vi "CSMStandApp.vi"() -> ()   [LabVIEW 2020, in "CSMStand-Engine(Lite).lvlib"]
doc: "------------- lvcsm -------------\n[CSMStates]\nItem 0 = \"Event Structure\"\nItem 1 = \"Idle\"\nItem 2 = \"CSM Documentation\"\nItem 3 = \"Error Handler\"\nItem 4 = \"VI Reference\"\nItem 5 = \"Critical Error\"\nItem 6 = \"Target Timeout Error\"\nItem 7 = \"Target Error\"\nItem 8 = \"Async Response\"\nItem 9 = \"Response\"\nItem 10 = \"Async Message Posted\"\nItem 11 = \"Initialize Core Data\"\nItem 12 = \"Exit\"\nItem 13 = \"Data: Initialize\"\nItem 14 = \"Data: Get Configuration\"\nItem 15 = \"Data: Get Internal Data\"\nItem 16 = \"Data: Set Configuration\"\nItem 17 = \"Data: Cleanup\"\nItem 18 = \"Events: Register\"\nItem 19 = \"Events: Unregister\"\nItem 20 = \"UI: Initialize\"\nItem 21 = \"UI: Cursor Set\"\nItem 22 = \"UI: Front Panel State\"\nItem 23 = \"UI: Insert CSMStand OI\"\nItem 24 = \"UI: Start CSMStand Engine Behind\"\nItem 25 = \"UI: Show Version Dialog\"\nItem 26 = \"UI: Update Title\"\nItem 27 = \"Macro: Initialize\"\nItem 28 = \"Macro: Exit\"\nItem 29 = \"API: Load Script File\"\nItem 30 = \"API: Unload Sequence File\"\nItem 31 = \"API: Information\"\nItem 32 = \"API: Settings\"\n\n[CSMStatus]\nItem 0 = \"Error Occurred@Error Handler\""
uses:
  f71e1bc3-10f1-4d1d-8987-c57c60744672.vi
  5479b9e0-3b99-47d2-9fb2-6b1a6c6fc50e.vi
  48aabd89-37f9-4145-9c04-d0fd28b441f4.vi
  35608a63-0d23-4e3c-87b1-9318b6aa47ba.vi
  1ae25337-ae93-478f-b23d-9afa4476f43f.vi
  <userlib>/_NEVSTOP/Communicable State Machine(CSM)/AdvanceAPI/CSM - Revert Arguments-Safe String.vi
  <userlib>/_NEVSTOP/Communicable State Machine(CSM)/AdvanceAPI/CSM - Break Down Multiple States String.vi
  <userlib>/_NEVSTOP/Communicable State Machine(CSM)/AdvanceAPI/CSM - Compact Multiple States.vi
  <userlib>/_NEVSTOP/Communicable State Machine(CSM)/AdvanceAPI/CSM - Keywords.vi
  <userlib>/_NEVSTOP/Communicable State Machine(CSM)/_Shared/Trim Single-line Text.vi
  <userlib>/_NEVSTOP/Communicable State Machine(CSM)/addons/API-String-Arugments-Support/_Support/Query Data as API String Arguments(variant).vi
  <userlib>/_NEVSTOP/Communicable State Machine(CSM)/addons/API-String-Arugments-Support/_Support/Convert API String Arguments to Data(variant).vi
  UI/ExecutionView(CSM).vi
  Engine/Engine(CSM).vi
  UI/VersionDialog(CSM).vi
  <userlib>/NEVSTOP-Programming-Palette/Dialog & Interface/Fit VI window to Caller Center_nevstop.vi
  <userlib>/_NEVSTOP/Communicable State Machine(CSM)/addons/API-String-Arugments-Support/_Support/Data To API String Arguments.vi
  <userlib>/_NEVSTOP/Communicable State Machine(CSM)/addons/MassData-Parameter/_support/FGV-MassData(lvlibp).vi
  CSMStand-Engine(Lite).lvlib
  <userlib>/_NEVSTOP/Communicable State Machine(CSM)/Communicable State Machine.lvlib
  <userlib>/_NEVSTOP/Communicable State Machine(CSM)/_tool/_ui/csm-ui-support.lvlib
  <userlib>/_NEVSTOP/Communicable State Machine(CSM)/addons/API-String-Arugments-Support/API String Arguments Support.lvlib
  <userlib>/_NEVSTOP/Communicable State Machine(CSM)/_tool/_file/csm-file-support.lvlib
panel:
  in  "Toolbar.Unload Script File":bool
  in  "Toolbar.Information":bool
  in  "Toolbar.Load Script File":bool
  in  "Toolbar.Terminate":bool
  in  "Toolbar.SinglePass":bool
  out "LOG":string
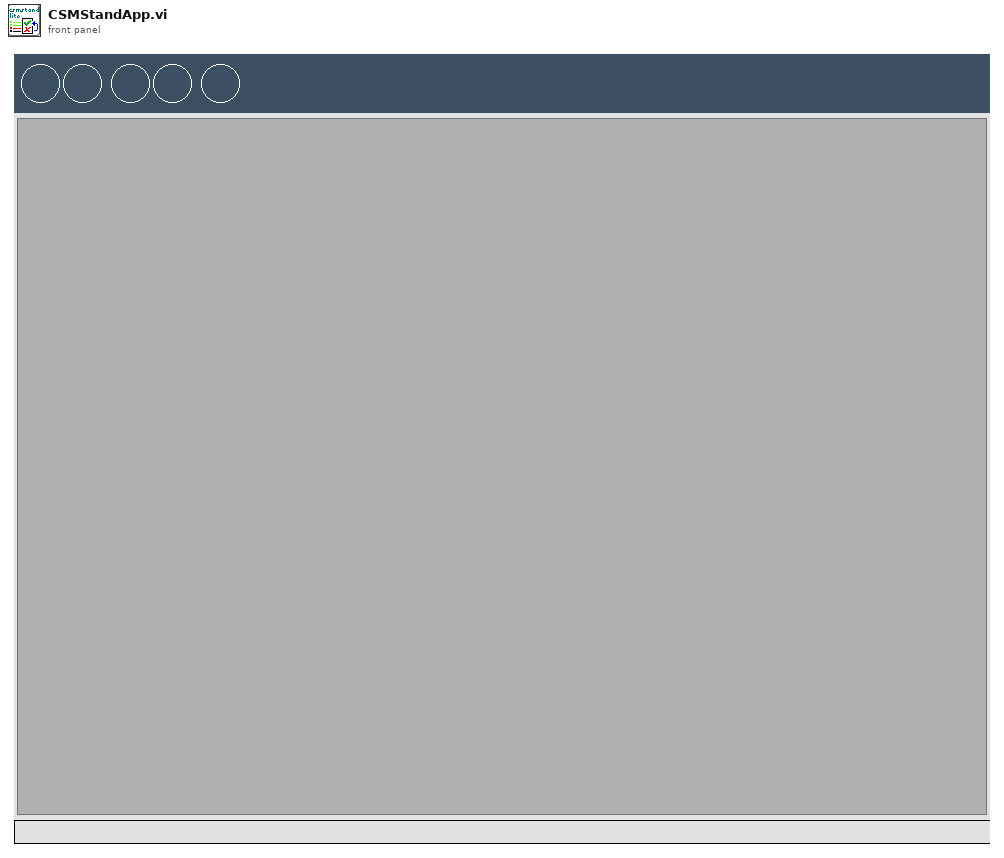
[diagram p1: front panel]
types:
  T1 = enum32{"Invalid", "Standard", "Closed", "Hidden", "Minimized", "Maximized"}
  T2 = enum32{"invalid app kind", "Development System", "Run Time System", "Student Edition", "Embedded LabVIEW", "Evaluation", "Custom"}
  T3 = typedef "Communicable State Machine.lvlib/_CSM_Response Source Message.ctl" = cluster{"‘State":string, "’Arguments":string, "’Error":errorcluster}
  T4 = cluster{"Current VI Reference":refnum<vi>, "Close Panel on Exit?":bool}
  T5 = cluster{"Core":cluster{"Current VI Reference":refnum<vi>, "Close Panel on Exit?":bool}, "DataBool":bool, "DataString":string, "Settings":cluster{"Boolean":bool, "string":string}}
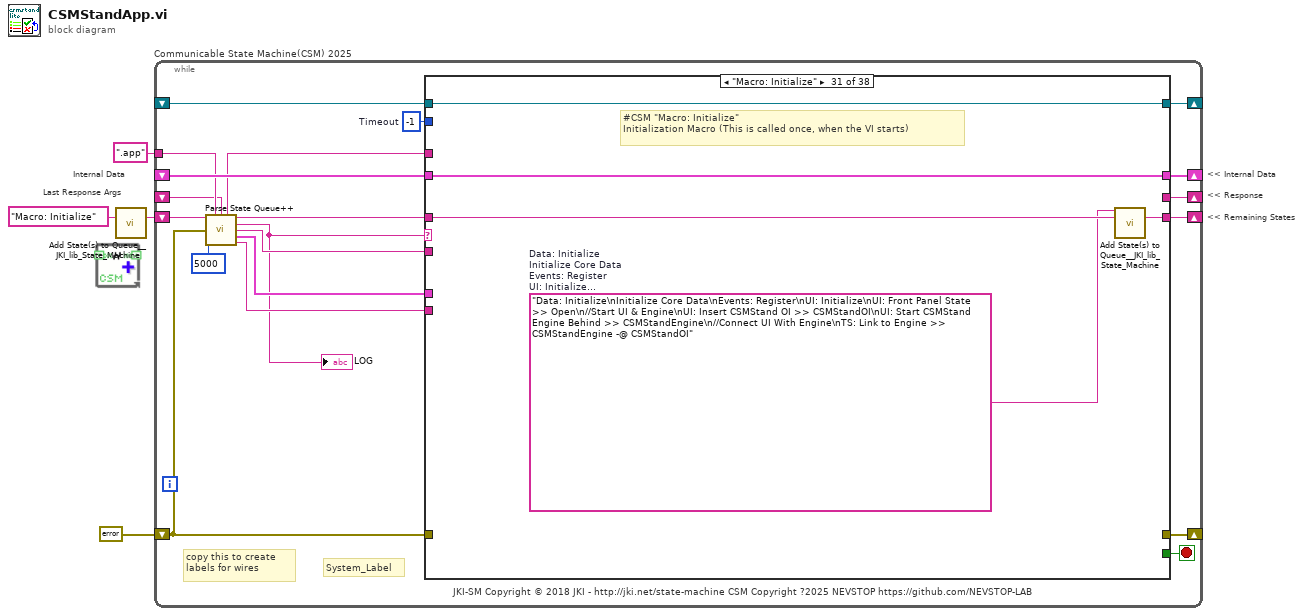
[diagram p0: block diagram]
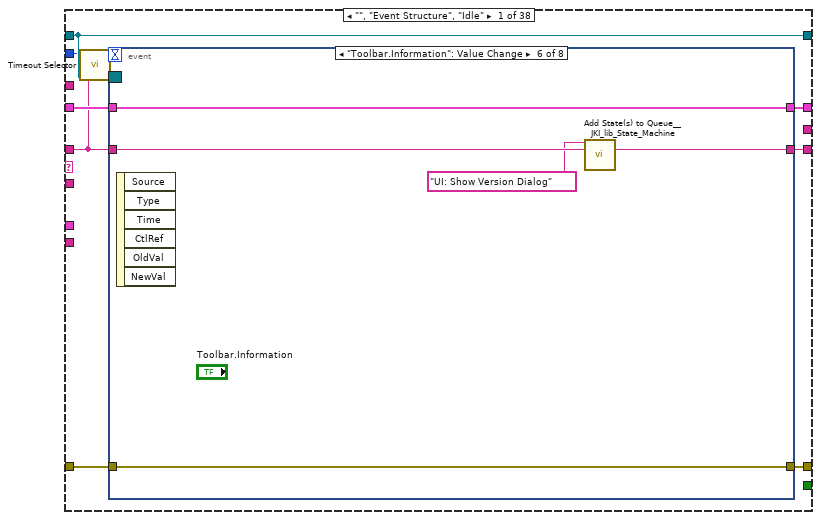
[diagram p2: hidden frame]
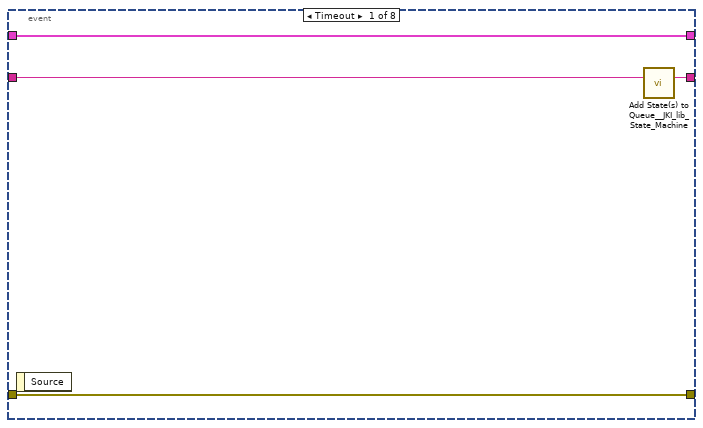
[diagram p3: hidden frame]
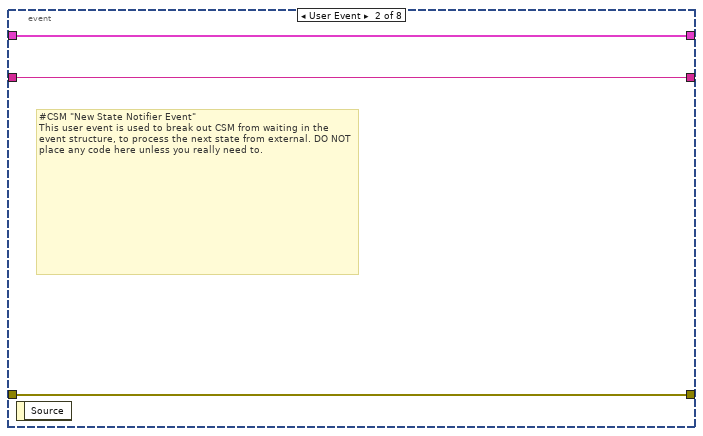
[diagram p4: hidden frame]
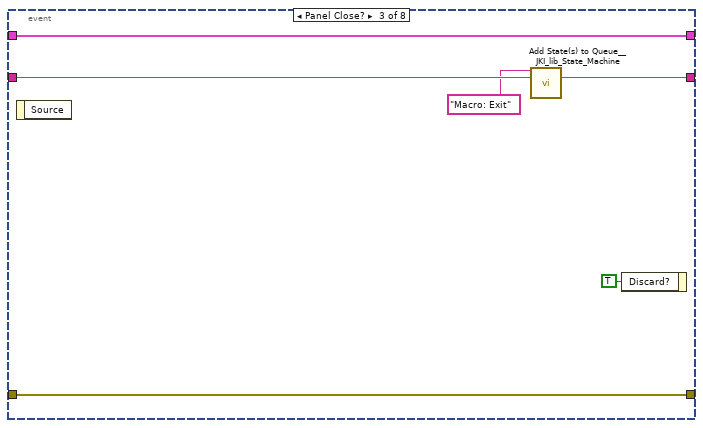
[diagram p5: hidden frame]
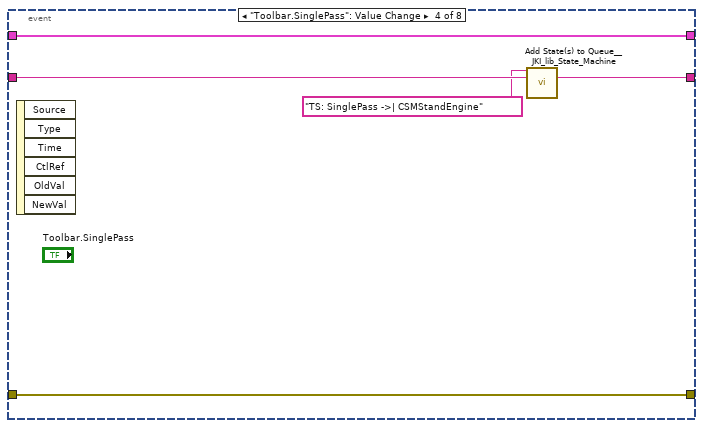
[diagram p6: hidden frame]
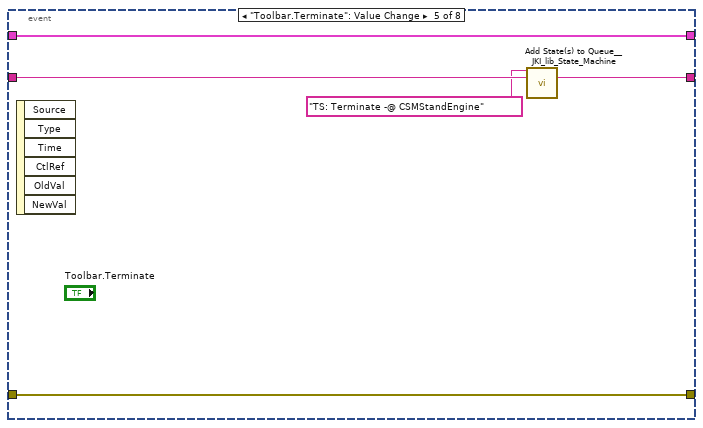
[diagram p7: hidden frame]
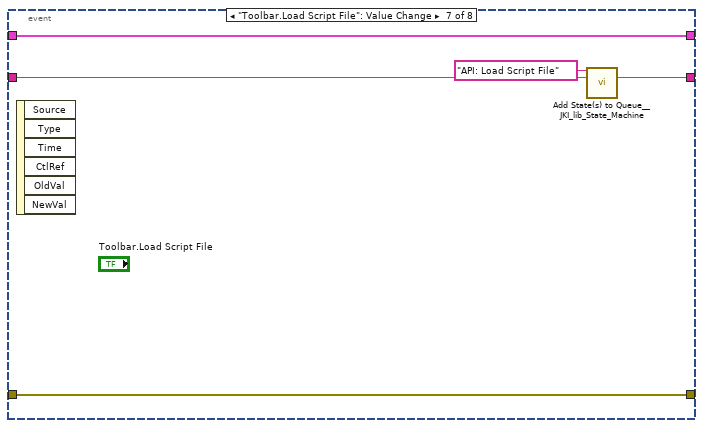
[diagram p8: hidden frame]
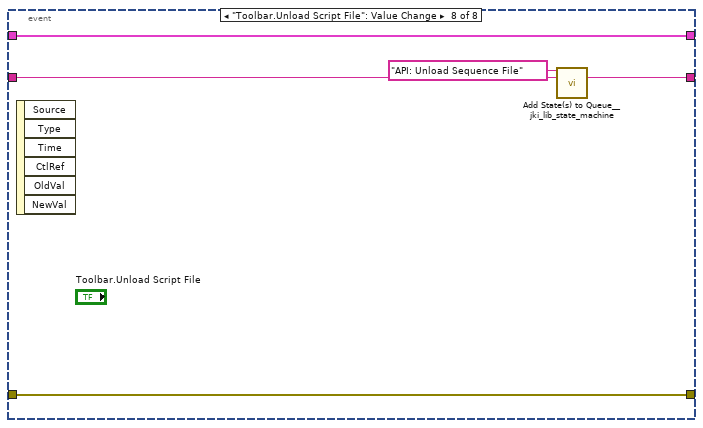
[diagram p9: hidden frame]
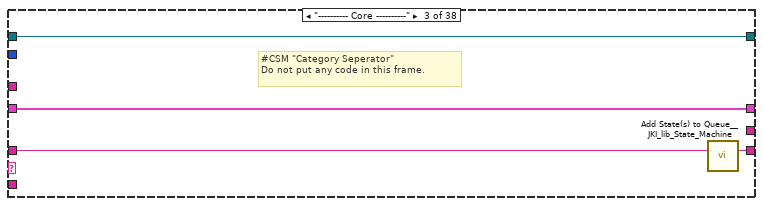
[diagram p11: hidden frame]
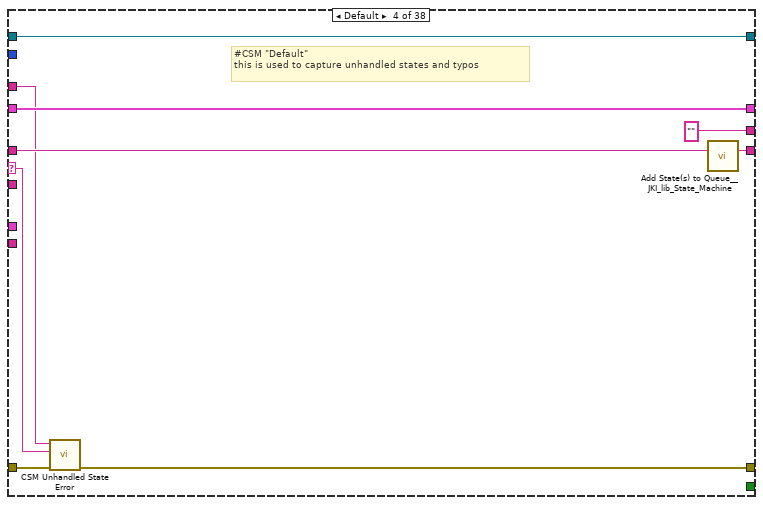
[diagram p12: hidden frame]
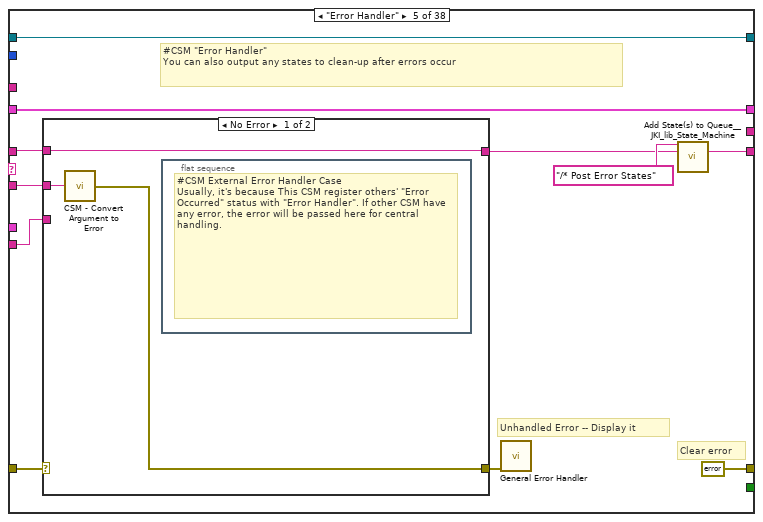
[diagram p13: hidden frame]
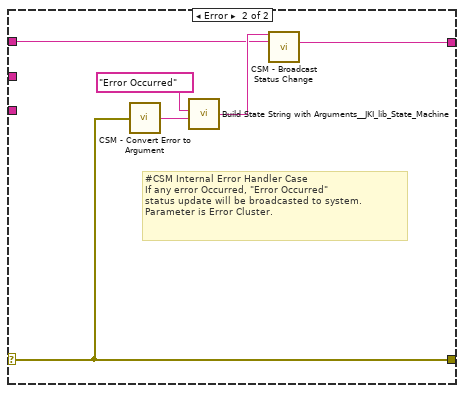
[diagram p14: hidden frame]
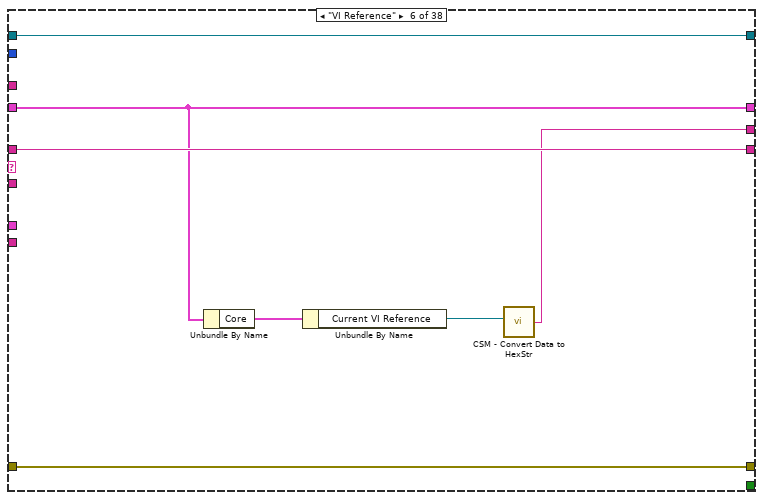
[diagram p15: hidden frame]
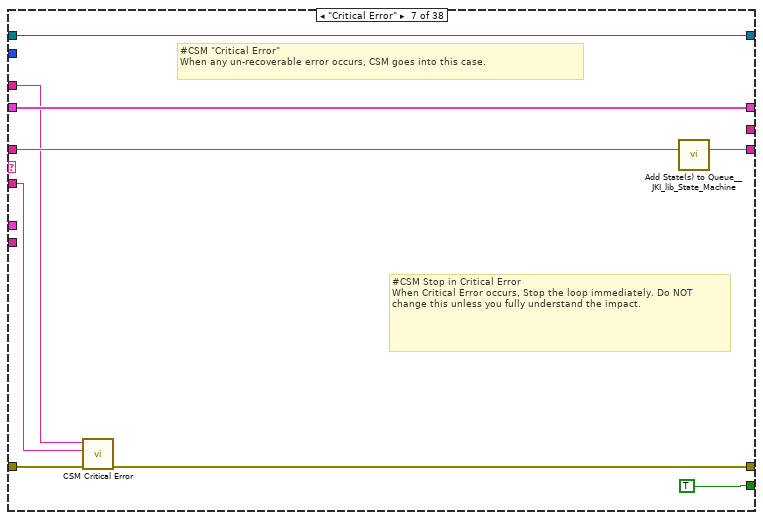
[diagram p16: hidden frame]
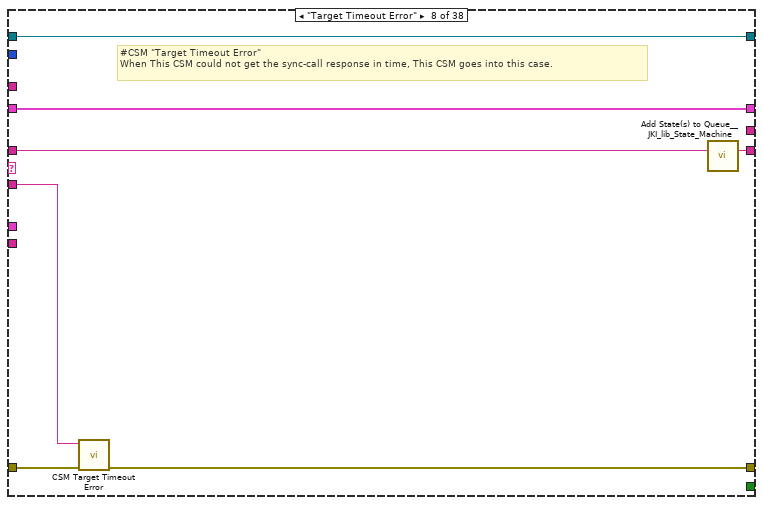
[diagram p17: hidden frame]
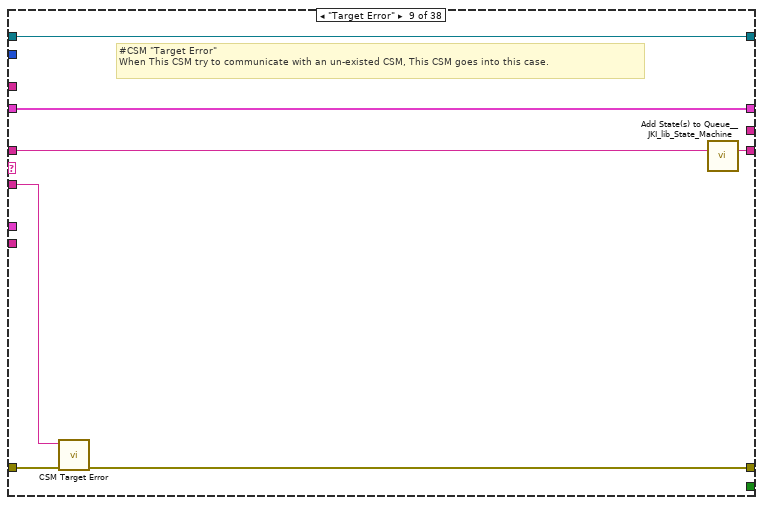
[diagram p18: hidden frame]
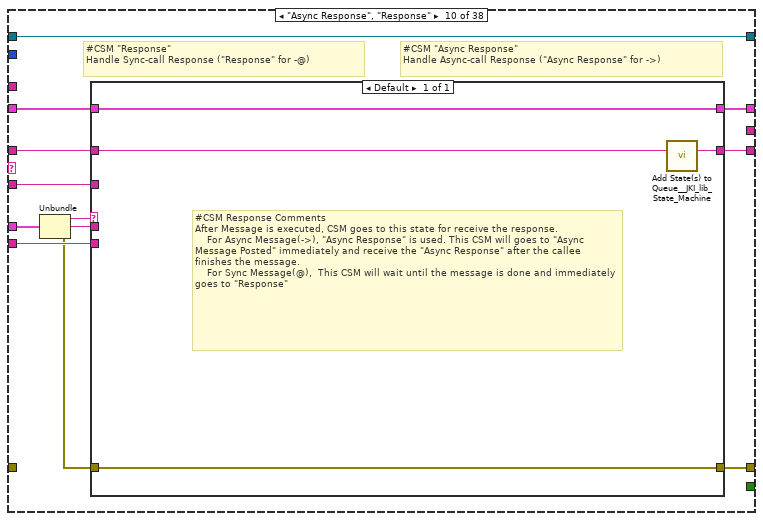
[diagram p19: hidden frame]
diagram:
  # "Last Response Args"
  # "Internal Data"
  # "<< Internal Data"
  # "<< Response"
  # "<< Remaining States"
  n1 = call <vilib>:"Add State(s) to Queue__JKI_lib_State_Machine.vi"("State(s) in (\"\")"="Macro: Initialize" ("Init States(\"Macro: Initialize\")")) -> ("States Out"=w3:string)  [unwired: 14 in]
  n2 = while "Communicable State Machine(CSM) 2025" {
    shift-right: [w19] -> _
    shift-left: _ -> [w18]
    shift-right: [w22] -> _
    shift-left: errorcluster {"status"=FALSE, "code"=0, "source"=""} ("error out") -> [w16]
    shift-right: [w21] -> _
    shift-left: w3 -> [w23]
    tunnel: ".app" ("Name(\"\" to use uuid)") -> [w11]
    shift-right: [w14] -> _
    shift-left: _ -> [w7]
    shift-right: [w13] -> _
    shift-left: _ -> [w12]
    stop <- w20 stop-if-true
    w17 = -1  # Timeout
    # "copy this to create labels for wires"
    # "System_Label"
    # "JKI-SM Copyright © 2018 JKI - http://jki.net/state-machine CSM Copyright ?2025 NEVSTOP https://github.com/NEVSTOP-LAB"
    n3 = call <userlib>:"Parse State Queue++.vi"("State Queue"=w23, "Name (\"\" to Use UUID)"=w11, "Response Arguments"=w7, "Previous Error"=w16, "Response Timeout (-2 Use Global Settings)"=5000 ("Response Timeout(1000ms)")) -> ("Name Used"=w8:string, "Remaining States"=w24:string, "Current State"=w5:string, "Arguments"=w6:string, "Additional Information"=w10:T3, "Source CSM"=w9:string)  [unwired: 5 in]
    "LOG" <- w5
    n4 = case shown="\"Macro: Initialize\"" w5 {
      selector: w5 -> [_ _ _ w82 _ _ _ _ _ _ _ _ _ _ _ _ _ _ _ _ _ _ _ _ _ _ _ _ _ _ _ _ _ _ _ _ _ _]
      tunnel: w24 -> [w25 w74 w78 w85 w91 w113 w122 w129 w136 w142 w156 w169 w175 w179 w187 w194 w200 w206 w210 w217 w221 w225 w236 w243 w258 w339 w353 w371 w383 w388 w393 w409 w412 w418 w438 w445 w448 w452]
      tunnel: w6 -> [_ _ _ _ w89 _ w120 w126 w133 w143 _ _ _ _ _ w189 w198 _ _ _ _ _ _ w238 w253 w321 w340 _ w376 _ _ _ _ _ _ _ _ _]
      tunnel: w18 -> [w32 w73 w76 w83 w97 w109 w123 w127 w134 w141 w155 w163 w173 w177 _ w192 w197 w202 w208 w216 w220 w223 w234 w241 w255 w338 w352 w356 w381 w386 w391 w406 w411 w430 w441 w444 w447 w450]
      tunnel: [w31 _ _ w87 errorcluster {"status"=FALSE, "code"=0, "source"=""} ("error out") w114 w116 w124 w131 w146 _ _ w172 _ _ w190 w195 w203 _ w211 w219 _ _ w239 w256 w324 w341 w357 w384 _ _ w407 _ w420 w442 _ _ _] -> w22
      tunnel: w16 -> [w30 _ _ w86 w95 w114 w117 w130 w137 _ _ _ w172 _ _ _ _ _ _ _ _ _ _ w240 _ _ _ _ w384 _ _ w407 _ _ w442 _ _ _]
      tunnel: [w33 w74 w77 w84 w93 w113 w121 w128 w135 w139 w156 w168 w174 w178 w186 w194 w200 w205 w209 w217 w221 w224 w235 w242 w257 w339 w353 w371 w383 w387 w392 w408 w412 w419 w439 w445 w448 w451] -> w21
      tunnel: [_ _ _ _ _ _ TRUE _ _ _ _ _ TRUE _ _ _ _ _ _ _ _ _ _ _ _ _ _ _ _ _ _ _ _ _ _ _ _ _] -> w20
      tunnel: [w29 w73 w76 w83 w97 w109 w123 w127 w134 w140 w155 w167 w173 w177 w185 w188 w196 w202 w208 w216 w220 w223 w234 w241 w255 w338 w352 w356 w381 w386 w391 w406 w411 w430 w441 w444 w447 w450] -> w19
      tunnel: w17 -> [w27 _ _ _ _ _ _ _ _ _ _ _ _ _ _ _ _ _ _ _ _ _ _ _ _ _ _ _ _ _ _ _ _ _ _ _ _ _]
      tunnel: w9 -> [_ _ _ _ w88 _ _ _ _ w144 _ _ _ _ _ _ _ _ _ _ _ _ _ _ _ _ _ _ _ _ _ _ _ _ _ _ _ _]
      tunnel: w10 -> [_ _ _ _ _ _ _ _ _ w145 _ _ _ _ _ _ _ _ _ _ _ _ _ _ _ _ _ _ _ _ _ _ _ _ _ _ _ _]
      tunnel: [_ _ _ "" _ w108 _ _ _ _ _ _ _ _ _ w191 _ _ _ _ _ _ _ _ _ _ _ _ _ _ _ _ _ _ _ _ _ _] -> w14
      tunnel: [w28 w72 w75 w80 w96 w112 w118 w125 w132 w149 w154 w157 w170 w176 w181 w193 w199 w201 w207 w215 w218 w222 w233 w237 w252 w337 w351 w370 w382 w385 w389 w399 w410 w429 w440 w443 w446 w449] -> w13
      tunnel: w12 -> [w28 w72 w75 w80 w96 w112 w118 w125 w132 w149 w154 w157 w170 w176 w181 w193 w199 w201 w207 _ w218 w222 w233 w237 w252 w337 w351 w370 w382 w385 w389 w399 w410 w429 w440 w443 w446 w449]
      tunnel: w8 -> [_ _ _ w79 _ _ w115 _ _ _ _ _ _ _ _ _ _ _ _ w214 _ _ _ _ _ w319 _ _ _ _ _ w397 _ _ _ _ _ _]
      frame "", "Event Structure", "Idle" {
        n5 = call <userlib>:"Timeout Selector.vi"("Remaining States"=w25, "Timeout Expected"=w27) -> ("Timeout"=w26:i32)  [unwired: 5 in]
        n6 = event shown="[5] \"Toolbar.Information\": Value Change" {
          selector: w28 -> [_ _ _ _ _ _ _ _]
          dyn-events: _ -> [_ _ _ _ _ _ _ _]
          timeout: w26 -> [_ _ _ _ _ _ _ _]
          tunnel: w25 -> [w37 w39 w46 w48 w53 w58 w63 w68]
          tunnel: [w36 w39 w45 w49 w54 w59 w64 w69] -> w33
          tunnel: w32 -> [w34 w40 w43 w50 w55 w60 w65 w70]
          tunnel: [w35 w38 w44 w51 w56 w61 w66 w71] -> w31
          tunnel: w30 -> [w35 w38 w44 w51 w56 w61 w66 w71]
          tunnel: [w34 w40 w43 w50 w55 w60 w65 w70] -> w29
          event Timeout {
            n7 = event-data() -> ()  [unwired: 1 in, 1 out]
            n8 = call <vilib>:"Add State(s) to Queue__JKI_lib_State_Machine.vi"("State(s) in (\"\")"=w37) -> ("States Out"=w36:string)  [unwired: 14 in]
          }
          event User Event {
            # "#CSM \"New State Notifier Event\"\nThis user event is used to break out CSM from waiting in the event structure, to process the next state from external. DO NOT place any code here unless you really need to."
            n9 = event-data() -> ()  [unwired: 1 in, 1 out]
          }
          event Panel Close? {
            n10 = event-data() -> ()  [unwired: 1 in, 1 out]
            n11 = call <vilib>:"Add State(s) to Queue__JKI_lib_State_Machine.vi"("State(s) in Front (\"\")"="Macro: Exit", "State(s) in (\"\")"=w46) -> ("States Out"=w45:string)  [unwired: 13 in]
            n12 = event-data("Discard?"=TRUE) -> ()  [unwired: 1 in, 1 out]
          }
          event "Toolbar.SinglePass": Value Change {
            n13 = event-data() -> ()  [unwired: 1 in, 6 out]
            n14 = call <vilib>:"Add State(s) to Queue__JKI_lib_State_Machine.vi"("State(s) in Front (\"\")"="TS: SinglePass ->| CSMStandEngine" ("State(s) in Front (\"\")"), "State(s) in (\"\")"=w48) -> ("States Out"=w49:string)  [unwired: 13 in]
          }
          event "Toolbar.Terminate": Value Change {
            n15 = event-data() -> ()  [unwired: 1 in, 6 out]
            n16 = call <vilib>:"Add State(s) to Queue__JKI_lib_State_Machine.vi"("State(s) in Front (\"\")"="TS: Terminate -@ CSMStandEngine" ("State(s) in Front (\"\")"), "State(s) in (\"\")"=w53) -> ("States Out"=w54:string)  [unwired: 13 in]
          }
          event "Toolbar.Information": Value Change {
            n17 = event-data() -> ()  [unwired: 1 in, 6 out]
            n18 = call <vilib>:"Add State(s) to Queue__JKI_lib_State_Machine.vi"("State(s) in Front (\"\")"="UI: Show Version Dialog" ("State(s) in Front (\"\")"), "State(s) in (\"\")"=w58) -> ("States Out"=w59:string)  [unwired: 13 in]
          }
          event "Toolbar.Load Script File": Value Change {
            n19 = event-data() -> ()  [unwired: 1 in, 6 out]
            n20 = call <vilib>:"Add State(s) to Queue__JKI_lib_State_Machine.vi"("State(s) in Front (\"\")"="API: Load Script File" ("State(s) in Front (\"\")"), "State(s) in (\"\")"=w63) -> ("States Out"=w64:string)  [unwired: 13 in]
          }
          event "Toolbar.Unload Script File": Value Change {
            n21 = event-data() -> ()  [unwired: 1 in, 6 out]
            n22 = call <vilib>:"Add State(s) to Queue__jki_lib_state_machine.vi"("State(s) in Front (\"\")"="API: Unload Sequence File" ("State(s) in Front (\"\")"), "State(s) in (\"\")"=w68) -> ("States Out"=w69:string)  [unwired: 13 in]
          }
        }
      }
      frame "CSM Documentation" {
        # "#CSM State Syntax\n\n// Comment line, all text to the right of “//” will be ignored\n// Local Message Example\nDoSth: DoA >> Arguments\n\n// Sync Call Example\nAPI: xxxx >> Arguments -@ TargetModule\n\n// Async Call Example\nAPI: xxxx >> Arguments -> TargetModule\n\n// Async Call without Reply Example\nAPI: xxxx >> Arguments ->| TargetModule\n\n// Broadcast normal status:\nStatus >> StatusArguments  -><status>\n\n// Broadcast Interrupt status:\nInterrupt >> StatusArguments  -><interrupt>\n\n// Register Source Module's status to Handler Module\nStatus@Source Module >> Handler Module@Handler Module -><register>\n\n// Unegister Source Module's status\nStatus@Source Module >> Handler Module -><unregister>"
        # "#CSM README FIRST\n\nCommunicable State Machine(CSM) is a LabVIEW application framework that builds upon JKI State Machine(JKISM). It follows the pattern of JKISM and extends the keywords to describe message communication between modules, including concepts such as Sync-Message, Async-Message, Subscription/Unsubscription of status - essential elements for creating reusable code modules. For more information, please visit the CSM wiki: https://nevstop-lab.github.io/CSM-Wiki/\n\nFor instructions on JKI State Machine, visit: \n    http://jki.net/state-machine/\nFor information about CSM, visit: \n    https://github.com/NEVSTOP-LAB"
        # "#CSM \"Documentation\"\nCase for holding CSM Documenation"
      }
      frame "---------- Core ----------" {
        # "#CSM \"Category Seperator\"\nDo not put any code in this frame."
        n23 = call <vilib>:"Add State(s) to Queue__JKI_lib_State_Machine.vi"("State(s) in (\"\")"=w78) -> ("States Out"=w77:string)  [unwired: 14 in]
      }
      frame Default {
        # "#CSM \"Default\"\nthis is used to capture unhandled states and typos"
        n24 = call <userlib>:"CSM Unhandled State Error.vi"("error in (no error)"=w86, "Undefined State"=w82, "CSM Name"=w79) -> ("error out"=w87:errorcluster)  [unwired: 8 in]
        n25 = call <vilib>:"Add State(s) to Queue__JKI_lib_State_Machine.vi"("State(s) in (\"\")"=w85) -> ("States Out"=w84:string)  [unwired: 14 in]
      }
      frame "Error Handler" {
        # "Unhandled Error -- Display it"
        # "#CSM \"Error Handler\"\nYou can also output any states to clean-up after errors occur"
        # "Clear error"
        n26 = case shown="No Error" w95 {
          selector: w95 -> [_ w102]
          tunnel: [w100 w104] -> w92
          tunnel: w91 -> [w100 w103]
          tunnel: [w99 w102] -> w90
          tunnel: w89 -> [w101 _]
          tunnel: w88 -> [_ _]
          frame No Error {
            n27 = call <userlib>:"CSM - Convert Argument to Error.vi"("Argument"=w101) -> ("Error"=w99:errorcluster)  [unwired: 4 in]
            n28 = flat-sequence {
              frame #0 {
                # "#CSM External Error Handler Case\nUsually, it's because This CSM register others' \"Error Occurred\" status with \"Error Handler\". If other CSM have any error, the error will be passed here for central handling."
              }
            }
          }
          frame Error {
            # "#CSM Internal Error Handler Case \nIf any error Occurred, \"Error Occurred\" \nstatus update will be broadcasted to system.\nParameter is Error Cluster."
            n29 = call <userlib>:"CSM - Convert Error to Argument.vi"("Error"=w102) -> ("Argument"=w106:string)  [unwired: 4 in]
            n30 = call <vilib>:"Build State String with Arguments__JKI_lib_State_Machine.vi"("Arguments (\"\")"=w106, "State"="Error Occurred" ("Status with Arguments")) -> ("State with Arguments"=w105:string)  [unwired: 4 in]
            n31 = call <userlib>:"CSM - Broadcast Status Change.vi"("Status With Arguments"=w105, "State Queue"=w103) -> ("Remaining States"=w104:string)  [unwired: 13 in]
          }
        }
        n32 = call <vilib>:"General Error Handler.vi"("error in (no error)"=w90) -> ()  [unwired: 10 in, 5 out]
        n33 = call <vilib>:"Add State(s) to Queue__JKI_lib_State_Machine.vi"("State(s) in Front (\"\")"="/* Post Error States", "State(s) in (\"\")"=w92) -> ("States Out"=w93:string)  [unwired: 13 in]
      }
      frame "VI Reference" {
        n34 = Unbundle By Name(w109) -> ("Core"=w111:T4)
        n35 = Unbundle By Name(w111) -> ("Current VI Reference"=w110:refnum<vi>)
        n36 = call <userlib>:"CSM - Convert Data to HexStr.vi"("Variant"=w110) -> ("HEX String (0-9,A-F)"=w108:string)  [unwired: 8 in]
      }
      frame "Critical Error" {
        # "#CSM \"Critical Error\"\nWhen any un-recoverable error occurs, CSM goes into this case."
        # "#CSM Stop in Critical Error\nWhen Critical Error occurs, Stop the loop immediately. Do NOT change this unless you fully understand the impact."
        n37 = call <userlib>:"CSM Critical Error.vi"("error in (no error)"=w117, "Arugments (As Reason)"=w120, "CSM Name"=w115) -> ("error out"=w116:errorcluster)  [unwired: 8 in]
        n38 = call <vilib>:"Add State(s) to Queue__JKI_lib_State_Machine.vi"("State(s) in (\"\")"=w122) -> ("States Out"=w121:string)  [unwired: 14 in]
      }
      frame "Target Timeout Error" {
        # "#CSM \"Target Timeout Error\"\nWhen This CSM could not get the sync-call response in time, This CSM goes into this case."
        n39 = call <userlib>:"CSM Target Timeout Error.vi"("error in (no error)"=w130, "Arguments (As CSM Name)"=w126) -> ("error out"=w124:errorcluster)  [unwired: 9 in]
        n40 = call <vilib>:"Add State(s) to Queue__JKI_lib_State_Machine.vi"("State(s) in (\"\")"=w129) -> ("States Out"=w128:string)  [unwired: 14 in]
      }
      frame "Target Error" {
        # "#CSM \"Target Error\"\nWhen This CSM try to communicate with an un-existed CSM, This CSM goes into this case."
        n41 = call <userlib>:"CSM Target Error.vi"("error in (no error)"=w137, "Arguments (As CSM Name)"=w133) -> ("error out"=w131:errorcluster)  [unwired: 9 in]
        n42 = call <vilib>:"Add State(s) to Queue__JKI_lib_State_Machine.vi"("State(s) in (\"\")"=w136) -> ("States Out"=w135:string)  [unwired: 14 in]
      }
      frame "Async Response", "Response" {
        # "#CSM \"Async Response\"\nHandle Async-call Response (\"Async Response\" for ->)"
        # "#CSM \"Response\"\nHandle Sync-call Response (\"Response\" for -@)"
        n43 = Unbundle(w145) -> ("‘State"=w148:string, "’Arguments"=w147:string, "’Error"=w138:errorcluster)
        n44 = case shown="Default" w148 {
          tunnel: [w150] -> w139
          tunnel: w142 -> [w151]
          tunnel: [w153] -> w140
          tunnel: w141 -> [w153]
          tunnel: [w152] -> w146
          tunnel: w138 -> [w152]
          tunnel: w144 -> [_]
          tunnel: w143 -> [_]
          tunnel: w147 -> [_]
          frame Default {
            # "#CSM Response Comments\nAfter Message is executed, CSM goes to this state for receive the response.\n    For Async Message(->), \"Async Response\" is used. This CSM will goes to \"Async Message Posted\" immediately and receive the \"Async Response\" after the callee finishes the message.\n    For Sync Message(@),  This CSM will wait until the message is done and immediately goes to \"Response\""
            n45 = call <vilib>:"Add State(s) to Queue__JKI_lib_State_Machine.vi"("State(s) in (\"\")"=w151) -> ("States Out"=w150:string)  [unwired: 14 in]
          }
        }
      }
      frame "Async Message Posted" {
        # "#CSM \"Async Message Posted\"\nAfter Async Message is posted (-> or ->| ), CSM goes to this state for post-action.\nYou can use Argument - State to tell which Async Message is called."
      }
      frame "Initialize Core Data" {
        # "#CSM \"Initialize Core Data\"\nThis is used to determine panel behavior on exit"
        # "originally closed?"
        # "exe?"
        # "If panel starts closed or is an EXE, then close it when we exit"
        n46 = property class="VI"() -> ("FP.State"=w160:T1)  [unwired: 2 in, 2 out]
        n47 = property class="App"() -> ("App.Kind"=w166:T2)  [unwired: 2 in, 2 out]
        n48 = control-ref of="Current VI Reference"() -> (w161:refnum<vi>)
        n49 = Equal?(x=w160, y=T1."Closed" ("Front Panel Window:State")) -> (x = y?=w158:bool)
        n50 = Equal?(x=w166, y=T2."Run Time System" ("Application:Kind")) -> (x = y?=w164:bool)
        n51 = Or(x=w158, y=w164) -> (x .or. y?=w162:bool)
        n52 = Bundle By Name(cluster=w163, "Core.Current VI Reference"=w161, "Core.Close Panel on Exit?"=w162) -> (w167:T5)
        n53 = call <vilib>:"Add State(s) to Queue__JKI_lib_State_Machine.vi"("State(s) in (\"\")"=w169) -> ("States Out"=w168:string)  [unwired: 14 in]
      }
      frame "Exit" {
        # "#CSM \"Exit\"\nCase for exiting the loop. No errors that occur here will be handled."
        n54 = call <vilib>:"Add State(s) to Queue__JKI_lib_State_Machine.vi"("State(s) in (\"\")"=w175) -> ("States Out"=w174:string)  [unwired: 14 in]
      }
      frame "---------- Data ----------" {
        # "#CSM \"Category Seperator\"\nDo not put any code in this frame."
        n55 = call <vilib>:"Add State(s) to Queue__JKI_lib_State_Machine.vi"("State(s) in (\"\")"=w179) -> ("States Out"=w178:string)  [unwired: 14 in]
      }
      frame "Data: Initialize" {
        w180 = cluster{"Boolean":bool, "string":string} {"Boolean"=TRUE, "string"=""}  # Settings
        w182 = T4 {"Current VI Reference"=refnum, "Close Panel on Exit?"=FALSE}  # Core
        w184 = TRUE  # DataBool
        w183 = ""  # DataString
        # "Expand Bundle to add new data elements to shift register data."
        # "Data names and types of shift register data are defined by this bundle."
        # "do not delete - used by framework"
        # "#CSM \"Data: Initialize\"\nInitialize the shift-register data, here.\n(data names are defined by what you wire into the bundle function)"
        n56 = Bundle("Core"=w182, "DataBool"=w184, "DataString"=w183, "Settings"=w180) -> (w185:T5)  [unwired: 1 in]
        n57 = call <vilib>:"Add State(s) to Queue__JKI_lib_State_Machine.vi"("State(s) in (\"\")"=w187) -> ("States Out"=w186:string)  [unwired: 14 in]
      }
      frame "Data: Get Configuration", "Data: Get Internal Data" {
        n58 = call "Query Data as API String Arguments.vim"("Name"=w189, "Cluster Data"=w192) -> ("error"=w190:errorcluster, "API String"=w191:string, "Cluster Data (dup)"=w188:T5)  [unwired: 7 in]
      }
      frame "Data: Set Configuration" {
        n59 = call "Convert API String Arguments to Data.vim"("Reference Type"=w197, "API String"=w198) -> ("error out"=w195:errorcluster, "Data"=w196:T5)  [unwired: 6 in]
      }
      frame "Data: Cleanup" {
        # "#CSM \"Data: Cleanup\"\nCleanup any data and references, here.\n(this is called automatically, by the Macro: Exit)"
        n60 = Unbundle By Name(w202) -> ("Core.Current VI Reference"=w204:refnum<vi>)
        n61 = Close Reference(reference=w204) -> (error out=w203:errorcluster)  [unwired: 1 in]
        n62 = call <vilib>:"Add State(s) to Queue__JKI_lib_State_Machine.vi"("State(s) in (\"\")"=w206) -> ("States Out"=w205:string)  [unwired: 14 in]
      }
      frame "---------- Events ----------" {
        # "#CSM \"Category Seperator\"\nDo not put any code in this frame."
        n63 = call <vilib>:"Add State(s) to Queue__JKI_lib_State_Machine.vi"("State(s) in (\"\")"=w210) -> ("States Out"=w209:string)  [unwired: 14 in]
      }
      frame "Events: Register" {
        # "#CSM \"Events: Register\"\nRegister user event. New Message Event is registered to break CSM waiting in event structure by default."
        # "#CSM Register New Message Event\nRegister message event to break Waiting in Event structure."
        n64 = call <userlib>:"CSM - Get New State Notifier Event.vi"("Name (\"\" to Use UUID)"=w214) -> ("error out"=w212:errorcluster, "New State Notifier Event"=w213:refnum<user-event>)  [unwired: 9 in]
        n65 = register-events(error in=w212, w213) -> (reference out=w215:refnum<event-registration>, error out=w211:errorcluster)  [unwired: 1 in]
      }
      frame "Events: Unregister" {
        # "#CSM \"Events: Unregister\"\nUnregister user event."
        n66 = Unregister For Events(event registration refnum=w218) -> (error out=w219:errorcluster)  [unwired: 1 in]
      }
      frame "---------- UI ----------" {
        # "#CSM \"Category Seperator\"\nDo not put any code in this frame."
        n67 = call <vilib>:"Add State(s) to Queue__JKI_lib_State_Machine.vi"("State(s) in (\"\")"=w225) -> ("States Out"=w224:string)  [unwired: 14 in]
      }
      frame "UI: Initialize" {
        # "#CSM \"UI: Initialize\"\nInitialize the User Interface, here.\n(this is called automatically, by the Macro: Init)"
        n68 = control-ref of="Toolbar.Load Script File"() -> (w228:refnum<vi>)
        n69 = control-ref of="Toolbar.Terminate"() -> (w229:refnum<vi>)
        n70 = control-ref of="Toolbar.SinglePass"() -> (w230:refnum<vi>)
        n71 = control-ref of="Toolbar.Information"() -> (w231:refnum<vi>)
        n72 = control-ref of="Splitter"() -> (w232:refnum<vi>)
        n73 = Build Array(w228, w229, w230, w231) -> (w227:refnum<vi>[])
        n74 = call <userlib>:"Relocate Splitter Posistion.vi"("Array"=w227, "Splitter in"=w232) -> ()  [unwired: 9 in, 1 out]
        n75 = call <vilib>:"Add State(s) to Queue__JKI_lib_State_Machine.vi"("State(s) in Front (\"\")"="UI: Update Title" ("State(s) in Front (\"\")"), "State(s) in (\"\")"=w236) -> ("States Out"=w235:string)  [unwired: 13 in]
      }
      frame "UI: Cursor Set" {
        # "Argument"
        # "#CSM \"UI: Cursor Set\"\nSet and Unset Cursor Busy.\n(Usage: \"UI: Cursor Set >> Busy|Idle\")"
        n76 = disable-structure shown="Default" {
          disable-tunnel: w240 -> [w246 w251]
          disable-tunnel: [w245 w251] -> w239
          disable-tunnel: w238 -> [w244 _]
          frame condition #0 (active) {
            n77 = case shown="\"Busy\"" w244 {
              tunnel: w246 -> [w248 w250]
              tunnel: [w247 w249] -> w245
              frame "Idle", Default {
                n78 = call <vilib>:"Unset Busy.vi"("error in (no error)"=w248) -> ("error out"=w247:errorcluster)  [unwired: 10 in]
              }
              frame "Busy" {
                n79 = call <vilib>:"Set Busy.vi"("error in (no error)"=w250) -> ("error out"=w249:errorcluster)  [unwired: 9 in, 1 out]
              }
            }
          }
          frame condition #1 {
          }
        }
        n80 = call <vilib>:"Add State(s) to Queue__JKI_lib_State_Machine.vi"("State(s) in (\"\")"=w243) -> ("States Out"=w242:string)  [unwired: 14 in]
      }
      frame "UI: Front Panel State" {
        # "Argument"
        # "#CSM \"UI: Front Panel State\"\nSet Front Panel Open or Closed\n(Usage: \"UI: Front Panel State >> Open|Close\")"
        n81 = Unbundle By Name(w255) -> ("Core.Current VI Reference"=w254:refnum<vi>)
        n82 = case shown="\"Minimize\", \"Minimized\"" w253 {
          tunnel: [w265 w278 w289 w301 w313] -> w256
          tunnel: w254 -> [w264 w276 w288 w300 w312]
          frame "Open", "Standard", Default {
            w259 = T1."Standard" ("State")
            n83 = property class="VI"(reference=w264) -> (reference out=w262:refnum<vi>, error out=w263:errorcluster, "FP.State"=w261:T1)  [unwired: 1 in]
            n84 = Not Equal?(x=w261, y=w259) -> (x != y?=w260:bool)
            n85 = case shown="True" w260 {
              tunnel: [w269 w271] -> w265
              tunnel: w263 -> [w268 w271]
              tunnel: w262 -> [w267 _]
              tunnel: w259 -> [w266 _]
              frame True {
                n86 = invoke class="VI" method="FP.Open"(reference=w267, error in=w268, "Activate"=TRUE, "State"=w266) -> (error out=w269:errorcluster)  [unwired: 1 in, 4 out]
              }
              frame False {
              }
            }
          }
          frame "Close", "Closed" {
            n87 = property class="VI"(reference=w276) -> (reference out=w275:refnum<vi>, error out=w277:errorcluster, "FP.State"=w273:T1)  [unwired: 1 in]
            n88 = Not Equal?(x=w273, y=T1."Closed" ("Front Panel Window:State")) -> (x != y?=w272:bool)
            n89 = case shown="True" w272 {
              tunnel: [w279 w282] -> w278
              tunnel: w277 -> [w279 w281]
              tunnel: w275 -> [_ w280]
              frame False {
              }
              frame True {
                n90 = invoke class="VI" method="FP.Close"(reference=w280, error in=w281) -> (error out=w282:errorcluster)  [unwired: 1 in, 2 out]
              }
            }
          }
          frame "Hidden", "Hide" {
            w283 = T1."Hidden" ("State")
            n91 = property class="VI"(reference=w288) -> (reference out=w286:refnum<vi>, error out=w287:errorcluster, "FP.State"=w285:T1)  [unwired: 1 in]
            n92 = Not Equal?(x=w285, y=w283) -> (x != y?=w284:bool)
            n93 = case shown="True" w284 {
              tunnel: [w293 w294] -> w289
              tunnel: w287 -> [w292 w294]
              tunnel: w286 -> [w291 _]
              tunnel: w283 -> [w290 _]
              frame True {
                n94 = invoke class="VI" method="FP.Open"(reference=w291, error in=w292, "State"=w290) -> (error out=w293:errorcluster)  [unwired: 2 in, 4 out]
              }
              frame False {
              }
            }
          }
          frame "Minimize", "Minimized" {
            w295 = T1."Minimized" ("State")
            n95 = property class="VI"(reference=w300) -> (reference out=w298:refnum<vi>, error out=w299:errorcluster, "FP.State"=w297:T1)  [unwired: 1 in]
            n96 = Not Equal?(x=w297, y=w295) -> (x != y?=w296:bool)
            n97 = case shown="False" w296 {
              tunnel: [w305 w306] -> w301
              tunnel: w299 -> [w304 w306]
              tunnel: w298 -> [w303 _]
              tunnel: w295 -> [w302 _]
              frame True {
                n98 = invoke class="VI" method="FP.Open"(reference=w303, error in=w304, "State"=w302) -> (error out=w305:errorcluster)  [unwired: 2 in, 4 out]
              }
              frame False {
              }
            }
          }
          frame "Maximize", "Maximized" {
            w307 = T1."Maximized" ("State")
            n99 = property class="VI"(reference=w312) -> (reference out=w310:refnum<vi>, error out=w311:errorcluster, "FP.State"=w309:T1)  [unwired: 1 in]
            n100 = Not Equal?(x=w309, y=w307) -> (x != y?=w308:bool)
            n101 = case shown="True" w308 {
              tunnel: [w317 w318] -> w313
              tunnel: w311 -> [w316 w318]
              tunnel: w310 -> [w315 _]
              tunnel: w307 -> [w314 _]
              frame True {
                n102 = invoke class="VI" method="FP.Open"(reference=w315, error in=w316, "State"=w314) -> (error out=w317:errorcluster)  [unwired: 2 in, 4 out]
              }
              frame False {
              }
            }
          }
        }
        n103 = call <vilib>:"Add State(s) to Queue__JKI_lib_State_Machine.vi"("State(s) in (\"\")"=w258) -> ("States Out"=w257:string)  [unwired: 14 in]
      }
      frame "UI: Insert CSMStand OI" {
        n104 = vi-ref "CSMStand-Engine(Lite).lvlib:ExecutionView(CSM).vi"() -> (w329:refnum<vi>)
        n105 = property class="VI (strict)"(reference=w329) -> (reference out=w333:refnum<vi>, error out=w331:errorcluster, "Path"=w330:path)  [unwired: 1 in]
        n106 = Open VI Reference(type specifier VI Refnum (for type only)=w333, vi path=w330, options=128, error in (no error)=w331) -> (vi reference=w332:refnum<vi>, error out=w328:errorcluster)  [unwired: 2 in]
        n107 = call-by-ref "Start Asynchronous Call"(reference=w332, error in=w328, "Name(\"\" to use uuid)"=w321) -> (reference out=w335:refnum<vi>, error out=w334:errorcluster)  [unwired: 11 in]
        n108 = Close Reference(reference=w335, error in (no error)=w334) -> (error out=w326:errorcluster)
        n109 = call <userlib>:"CSM - Wait for Module to Be Alive.vi"("CSM Name"=w321, "error in (no error)"=w326) -> ("CSM Name (Dup)"=w320:string, "error out"=w322:errorcluster)  [unwired: 11 in, 1 out]
        n110 = call <userlib>:"CSM - Module VI Reference.vi"("Current Module (\"\" to Generate an ID)"=w319, "error in (no error)"=w322, "Force? (F)"=TRUE, "CSM Name"=w320) -> ("error out"=w327:errorcluster, "CSM Module VIRef"=w325:refnum<vi>)  [unwired: 6 in]
        n111 = invoke on="Sub Panel" class="SubPnl" method="Insert VI"(error in=w327, "VI Ref"=w325) -> (error out=w324:errorcluster)  [unwired: 2 in, 3 out]
      }
      frame "UI: Start CSMStand Engine Behind" {
        n112 = vi-ref "CSMStand-Engine(Lite).lvlib:Engine(CSM).vi"() -> (w343:refnum<vi>)
        n113 = property class="VI (strict)"(reference=w343) -> (reference out=w347:refnum<vi>, error out=w345:errorcluster, "Path"=w344:path)  [unwired: 1 in]
        n114 = Open VI Reference(type specifier VI Refnum (for type only)=w347, vi path=w344, options=128, error in (no error)=w345) -> (vi reference=w346:refnum<vi>, error out=w342:errorcluster)  [unwired: 2 in]
        n115 = call-by-ref "Start Asynchronous Call"(reference=w346, error in=w342, "Name(\"\" to use uuid)"=w340) -> (reference out=w349:refnum<vi>, error out=w348:errorcluster)  [unwired: 11 in]
        n116 = Close Reference(reference=w349, error in (no error)=w348) -> (error out=w341:errorcluster)
      }
      frame "UI: Show Version Dialog" {
        w355 = "UI.VersionDlg" ("Name(\"\" to use uuid)")
        n117 = Unbundle By Name(w356) -> ("Core.Current VI Reference"=w354:refnum<vi>)
        n118 = vi-ref "CSMStand-Engine(Lite).lvlib:VersionDialog(CSM).vi"() -> (w362:refnum<vi>)
        n119 = property class="VI (strict)"(reference=w362) -> (reference out=w366:refnum<vi>, error out=w364:errorcluster, "Path"=w363:path)  [unwired: 1 in]
        n120 = Open VI Reference(type specifier VI Refnum (for type only)=w366, vi path=w363, options=128, error in (no error)=w364) -> (vi reference=w365:refnum<vi>, error out=w361:errorcluster)  [unwired: 2 in]
        n121 = call-by-ref "Start Asynchronous Call"(reference=w365, error in=w361, "Name(\"\" to use uuid)"=w355) -> (reference out=w368:refnum<vi>, error out=w367:errorcluster)  [unwired: 11 in]
        n122 = Close Reference(reference=w368, error in (no error)=w367) -> (error out=w360:errorcluster)
        n123 = call <userlib>:"CSM - Module VI Reference.vi"("error in (no error)"=w360, "CSM Name"=w355) -> ("error out"=w359:errorcluster, "CSM Module VIRef"=w358:refnum<vi>)  [unwired: 8 in]
        n124 = call-poly <userlib>:"Fit VI window_nevstop.vi"("Error In"=w359, "Background VI Ref (Callee's Caller)"=w354, "VI Ref (calling VI)"=w358) -> ("Error Out"=w357:errorcluster)  [unwired: 3 in, 1 out]
      }
      frame "UI: Update Title" {
        n125 = Unbundle By Name(w381) -> ("Core.Current VI Reference"=w380:refnum<vi>)
        n126 = call "Convert API String Arguments to Data.vim"("Reference Type"=path "", "API String"=w376) -> ("Data"=w375:path)  [unwired: 6 in, 1 out]
        n127 = Path To String(path=w375) -> (string=w373:string)
        n128 = call <userlib>:"Concatenate Strings If not Empty_csm.vi"("String"=w373, "seperator(:)"=" - ", "prefix"="CSMStand-Lite" ("Front Panel Window:Title")) -> ("result"=w379:string)  [unwired: 2 in]
        n129 = property class="VI"(reference=w380, "Front Panel.Title"=w379) -> (error out=w372:errorcluster)  [unwired: 1 in, 1 out]
        n130 = call <vilib>:"Clear Errors.vi"("error in (no error)"=w372) -> ()  [unwired: 5 in, 2 out]
      }
      frame "---------- Macro ----------" {
        # "#CSM \"Category Seperator\"\nDo not put any code in this frame."
        n131 = call <vilib>:"Add State(s) to Queue__JKI_lib_State_Machine.vi"("State(s) in (\"\")"=w388) -> ("States Out"=w387:string)  [unwired: 14 in]
      }
      frame "Macro: Initialize" {
        w390 = "Data: Initialize\nInitialize Core Data\nEvents: Register\nUI: Initialize\nUI: Front Panel State >> Open\n//Start UI & Engine\nUI: Insert CSMStand OI >> CSMStandOI\nUI: Start CSMStand Engine Behind >> CSMStandEngine\n//Connect UI With Engine\nTS: Link to Engine >> CSMStandEngine -@ CSMStandOI"  # Data: Initialize Initialize Core Data Events: Register UI: Initialize UI: Front Panel State >> Open //Start UI & Engine UI: Insert CSMStand OI >> CSMStandOI UI: Start CSMStand Engine Behind >> CSMStandEngine //Connect UI With Engine TS: Link to Engine >> CSMStandEngine -@ CSMStandOI
        # "#CSM \"Macro: Initialize\"\nInitialization Macro (This is called once, when the VI starts)"
        n132 = call <vilib>:"Add State(s) to Queue__JKI_lib_State_Machine.vi"("State(s) in Front (\"\")"=w390, "State(s) in (\"\")"=w393) -> ("States Out"=w392:string)  [unwired: 13 in]
      }
      frame "Macro: Exit" {
        w404 = "UI: Front Panel State >> Close"  # UI: Front Panel State >> Close
        # "#CSM \"Macro: Exit\"\nExit Macro (This is called once, when the VI exits)"
        n133 = Unbundle By Name(w406) -> ("Core.Close Panel on Exit?"=w405:bool)
        n134 = call <userlib>:"CSM - List Modules.vi"() -> ("Module Names"=w396:string[])  [unwired: 10 in, 1 out]
        n135 = Search 1D Array(1D array=w396, element=w397) -> (index of element=w394:i32)  [unwired: 1 in]
        n136 = Delete From Array(array=w396, index=w394) -> (array with subset deleted=w395:string[])  [unwired: 1 in, 1 out]
        n137 = Select(t=w404, s=w405, f="") -> (s? t:f=w402:string)
        n138 = call <userlib>:"CSM - Build Exit Messages of CSMs.vi"("CSMs"=w395) -> ("States"=w398:string)  [unwired: 14 in]
        n139 = call <vilib>:"Add State(s) to Queue__JKI_lib_State_Machine.vi"("State(s) in Front (\"\")"=w398, "State(s) in (\"\")"=w402, "State(s) at Back (\"\")"="Data: Cleanup\nEvents: Unregister\nExit") -> ("States Out"=w400:string)  [unwired: 12 in]
        n140 = call <vilib>:"Add State(s) to Queue__JKI_lib_State_Machine.vi"("State(s) in Front (\"\")"=w400, "State(s) in (\"\")"=w409) -> ("States Out"=w408:string)  [unwired: 13 in]
      }
      frame "---------- API ----------" {
        # "#CSM \"Category Seperator\"\nDo not put any code in this frame."
      }
      frame "API: Load Script File" {
        n141 = call "File Dialog"("pattern (all files)"="*.csmscript") -> ("selected path"=w414:path, "error out"=w427:errorcluster)  [unwired: 11 in, 2 out]
        n142 = Not A Number/Path/Refnum?(number/path/refnum=w414) -> (NaN/Path/Refnum?=w413:bool)
        n143 = call <userlib>:"TxtFile Load_CSM.vi"("error in (no error)"=w427, "Path"=w414) -> ("error out"=w421:errorcluster, "Text"=w426:string)  [unwired: 8 in]
        n144 = case shown="False" w413 {
          tunnel: [w436 _] -> w415
          tunnel: w414 -> [w435 _]
          frame False {
            n145 = call "Convert Data To API String Arguments.vim"("Data"=w435) -> ("API String"=w436:string)  [unwired: 7 in, 1 out]
          }
          frame True {
          }
        }
        n146 = disable-structure shown="Enabled" {
          disable-tunnel: w426 -> [w432 w434]
          disable-tunnel: [w431 w433] -> w425
          frame Disabled {
            n147 = call <userlib>:"CSM - Make String Arguments Safe.vi"("Argument String"=w432) -> ("Safe Argument String"=w431:string)  [unwired: 8 in]
          }
          frame Enabled {
            n148 = call "CSM - Convert MassData to Argument.vim"("Data"=w434) -> ("MassData Argument"=w433:string)  [unwired: 7 in, 1 out]
          }
        }
        n149 = call <vilib>:"Build State String with Arguments__JKI_lib_State_Machine.vi"("Arguments (\"\")"=w415, "State"="UI: Update Title" ("State(s) at Back (\"\")")) -> ("State with Arguments"=w417:string)  [unwired: 4 in]
        n150 = call <userlib>:"CSM - Send Message and Wait for Reply.vi"("Error In (No Error)"=w421, "Target Module"="CSMStandEngine", "Arguments (\"\")"=w425, "State"="TS: Load Sequence") -> ("error out"=w423:errorcluster)  [unwired: 5 in, 2 out]
        n151 = call <vilib>:"Clear Errors.vi"("error in (no error)"=w423) -> ("error out"=w420:errorcluster)  [unwired: 5 in, 1 out]
        n152 = call <vilib>:"Add State(s) to Queue__JKI_lib_State_Machine.vi"("State(s) in (\"\")"=w418, "State(s) at Back (\"\")"=w417) -> ("States Out"=w419:string)  [unwired: 13 in]
      }
      frame "API: Unload Sequence File" {
        n153 = call <vilib>:"Add State(s) to Queue__jki_lib_state_machine.vi"("State(s) in Front (\"\")"="TS: Unload Sequence ->| CSMStandEngine" ("State(s) in Front (\"\")"), "State(s) in (\"\")"=w438) -> ("States Out"=w439:string)  [unwired: 13 in]
      }
      frame "API: Information" {
      }
      frame "API: Settings" {
      }
      frame "---------- Action ----------" {
        # "#CSM \"Category Seperator\"\nDo not put any code in this frame."
        n154 = call <vilib>:"Add State(s) to Queue__JKI_lib_State_Machine.vi"("State(s) in (\"\")"=w452) -> ("States Out"=w451:string)  [unwired: 14 in]
      }
    }
  }
